vi "Read Map of Message Indexes to Write Info.vi"(8 "error in":errorcluster, 11 "Tx execution unit in":refnum<class "Tx Execution Unit.lvclass">) -> (0 "error out":errorcluster, 2 "map of message indexes to write info":T1, 3 "Tx execution unit out":refnum<class "Tx Execution Unit.lvclass">)   [LabVIEW 2020, in "AIM MIL-STD-1553 Engine.lvlib" / "Implementation.lvlib" / "Tx Execution Unit.lvclass"]
uses:
  Tx Execution Unit.lvclass
  Shared/Map of Message Indexes to Tx Write Info.ctl
  Shared/Tx Write Info.ctl
  Tx Execution Unit.lvclass/Tx Execution Unit.ctl
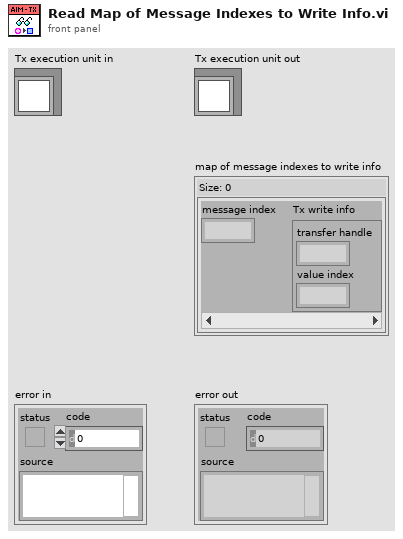
[diagram p1: front panel]
types:
  T1 = typedef "Map of Message Indexes to Tx Write Info.ctl" = map{i32, T2}
  T2 = typedef "Tx Write Info.ctl" = cluster{"transfer handle":u64, "value index":i32}
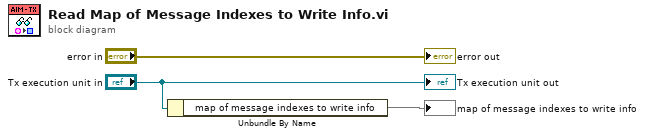
[diagram p0: block diagram]
diagram:
  n1 = Unbundle By Name("Tx execution unit in") -> ("map of message indexes to write info"=→"map of message indexes to write info":T1)
  "error out" <- "error in"
  "Tx execution unit out" <- "Tx execution unit in"
